vi "SmoothSurface.vi"(10 "Bit Depth":i32=8, 11 "Eye in":i16[][](array[numeric])) -> (3 "Smooth out":i16[][](array[numeric]))   [LabVIEW 2022 SP3]
uses:
  <vilib>/Analysis/NI_AALPro.lvlib
  <vilib>/Analysis/NI_AALBase.lvlib
panel:
  in  "initial Skip index":i32=50
  in  "Edge Thresh":i32=25
  in  "AS Med Fil":i32=10
  out "Overlay 2":dbl[][](graph)
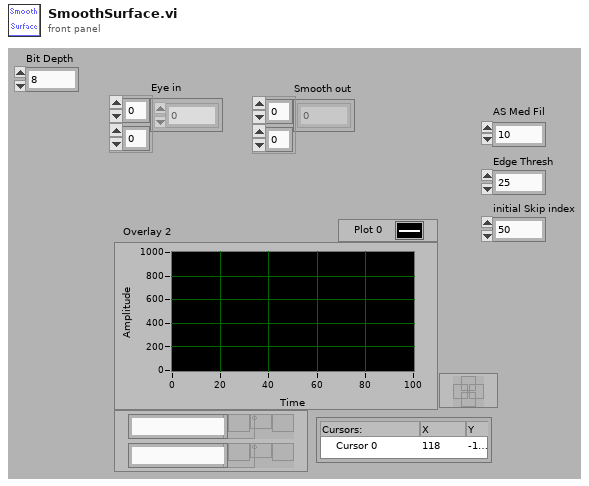
[diagram p1: front panel]
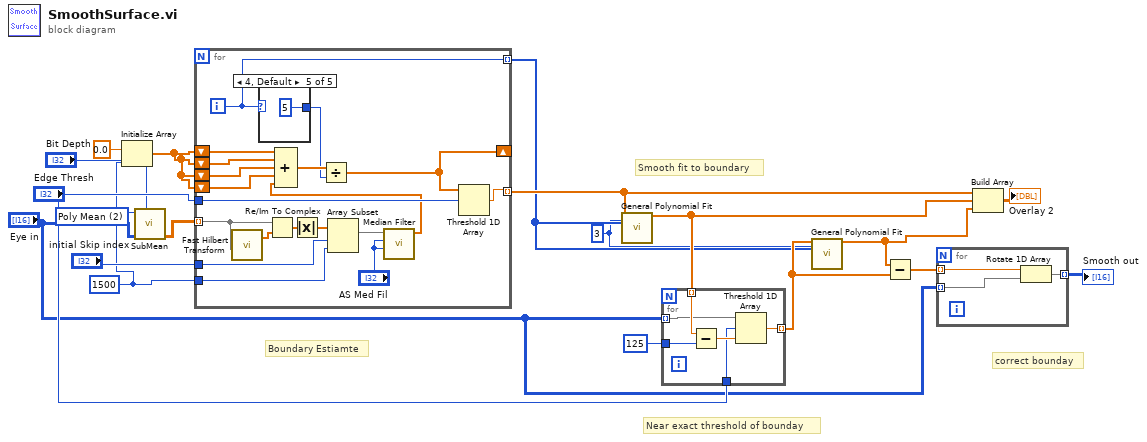
[diagram p0: block diagram]
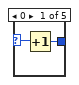
[diagram p2: hidden frame]
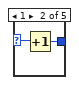
[diagram p3: hidden frame]
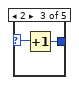
[diagram p4: hidden frame]
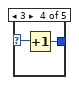
[diagram p5: hidden frame]
diagram:
  w2 = u16 2 items=["Mean from lines", "Mean just lines", "Poly Mean", "No mean"] ("Type of Mean")
  w7 = 1500
  w5 = 3
  # "correct bounday"
  # "Near exact threshold of bounday"
  # "Smooth fit to boundary"
  # "Boundary Estiamte"
  n1 = Initialize Array(0.0 ("element"), w7) -> (w6:dbl[])
  n2 = call "SubMean.vi"("Bit Depth"="Bit Depth", "Scan Data In"="Eye in", "Type of Mean"=w2) -> ("Array"=w4:dbl[][])  [unwired: 3 in, 2 out]
  n3 = for {
    tunnel: "Edge Thresh" -> [w31]
    tunnel: w4 -> [w30] mode=indexing
    shift-right: [w21] -> _
    shift-left: w6 -> [w38]
    shift-left: w6 -> [w37]
    shift-left: w6 -> [w35]
    tunnel: "initial Skip index" -> [w28]
    shift-left: w6 -> [w25]
    tunnel: w7 -> [w26]
    tunnel: [w24] -> w16 mode=indexing
    tunnel: [w20] -> w11 mode=indexing
    i -> [w20]
    n4 = call <vilib>:"Fast Hilbert Transform.vi"("X"=w30) -> ("Hilbert{X}"=w33:dbl[])  [unwired: 1 out]
    n5 = case shown="4, Default" w20 {
      selector: w20 -> [w40 w42 w44 w46 _]
      tunnel: [w39 w41 w43 w45 5] -> w32
      frame 0 {
        n6 = Increment(x=w40) -> (x+1=w39:i32)
      }
      frame 1 {
        n7 = Increment(x=w42) -> (x+1=w41:i32)
      }
      frame 2 {
        n8 = Increment(x=w44) -> (x+1=w43:i32)
      }
      frame 3 {
        n9 = Increment(x=w46) -> (x+1=w45:i32)
      }
      frame 4, Default {
      }
    }
    n10 = Re/Im To Complex(1:w33, 2:w30) -> (0:w34:cdb[])
    n11 = Absolute Value(x=w34) -> (abs(x)=w29:dbl[])
    n12 = Array Subset(array=w29, index=w28, length=w26) -> (w27:dbl[])
    n13 = call <vilib>:"Median Filter.vi"("right rank"="AS Med Fil", "left rank"="AS Med Fil", "X"=w27) -> ("Filtered X"=w22:dbl[])  [unwired: 8 out]
    n14 = Compound Arithmetic op=ADD(w38, w37, w35, w25, w22) -> (w36:dbl[])
    n15 = Divide(x=w36, y=w32) -> (x/y=w21:dbl[])
    n16 = Threshold 1D Array(2:w31, 3:w21) -> (0:w24:dbl)  [unwired: 1 out]
  }
  n17 = call <vilib>:"General Polynomial Fit.vi"("Y"=w16, "polynomial order"=w5, "X"=w11) -> ("Best Polynomial Fit"=w15:dbl[])  [unwired: 9 in, 3 out]
  n18 = for {
    tunnel: "Eye in" -> [w48] mode=indexing
    tunnel: 125 -> [w52]
    tunnel: [w51] -> w14 mode=indexing
    tunnel: w15 -> [w50] mode=indexing
    tunnel: "Edge Thresh" -> [w49]
    n19 = Subtract(x=w50, y=w52) -> (x-y=w53:dbl)
    n20 = Threshold 1D Array(1:w53, 2:w49, 3:w48) -> (0:w51:dbl)
  }
  n21 = call <vilib>:"General Polynomial Fit.vi"("Y"=w14, "polynomial order"=w5, "X"=w11) -> ("Best Polynomial Fit"=w10:dbl[])  [unwired: 9 in, 3 out]
  n22 = Subtract(x=w10, y=w14) -> (x-y=w13:dbl[])
  n23 = for {
    tunnel: [w56] -> w12 mode=indexing
    tunnel: w13 -> [w55] mode=indexing
    tunnel: "Eye in" -> [w54] mode=indexing
    n24 = Rotate 1D Array(1:w54, 2:w55) -> (0:w56:i16[])
  }
  "Smooth out" <- w12
  n25 = Build Array(w16, w15, w10) -> (→"Overlay 2":dbl[][])
